vi "Arcade Drive Translate.vi"(8 "xAxis":dbl, 9 "yAxis":dbl) -> (1 "outputX":dbl, 2 "outputY":dbl)   [LabVIEW 2015]
uses:
  Global Ref.vi
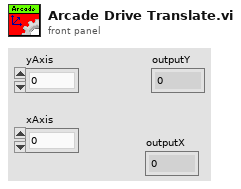
[diagram p1: front panel]
types:
  T1 = typedef "Global Ref typedef.ctl" = cluster{"Drive":cluster{"RobotDriveDevRef":T2}, "Joysticks":cluster{"JoyDriveRef":T10, "JoyOpRef":T10, "JoySabatourRef":T10}, "Lift":cluster{"LiftMotorRefLeft":T3, "LiftMotorRefRight":T3}, "Lift Limits":cluster{"Bottom Left":T12, "Bottom Right":T12}, "Accel":cluster{"AccelerometerDevRef":T14}, "Lift Encoder":cluster{"AIDeviceRefRight":T22, "AIDeviceRefLeft":T22}, "Lights":cluster{"Swag Light Ref cluster":cluster{"PWMDeviceRef1":T23, "PWMDeviceRef2":T23, "PWMDeviceRef3":T23, "PWMDeviceRef4":T23, "PWMDeviceRef5":T23, "PWMDeviceRef6":T23, "PWMDeviceRef7":T23, "PWMDeviceRef8":T23}}, "Camera":cluster{"GrayScaleImage":T24, "ColorImage":T24, "CameraDevRef":T25}, "Drive Encoders":cluster{"AIDeviceRef Left":T22, "AIDeviceRef Right":T22}, "Gyro":cluster{"GyroDevRef":T26}, "Relay":cluster{"RelayDevRef":T27, "RelayDevRef 2":T27}, "Gripper Arm Motors":cluster{"Gripper Arm Left":T3, "Gripper Arm Right":T3}, "Gripper Arm Limit":cluster{"Gripper Arm Left":T12, "Gripper Arm Right":T12}}
  T2 = typedef "WPI_RobotDriveDevRef.ctl" = cluster{"DevStatus":errorcluster, "Motors[]":T3[], "Square Inputs":bool, "Max Output":dbl}
  T3 = typedef "WPI_MotorControlDeviceRef.ctl" = cluster{"DeviceStatus":errorcluster, "Type":T4, "PWM":cluster{"PWM Channel":T5, "DeadBand":T6}, "CAN":cluster{"Device Number":u8, "Control Mode":T7, "Semaphore":T8, "Max Vout":dbl, "TalonSRX Control Mode":T9}, "Invert":bool}
  T4 = typedef "WPI_MotorControlType.ctl" = enum16{"PWM", "CAN", "CANTalonSRX"}
  T5 = typedef "FPGA_DIOPWMChannel.ctl" = enum8{"PWM 0", "PWM 1", "PWM 2", "PWM 3", "PWM 4", "PWM 5", "PWM 6", "PWM 7", "PWM 8", "PWM 9", "PWM MXP 0", "PWM MXP 1", "PWM MXP 2", "PWM MXP 3", "PWM MXP 4", "PWM MXP 5", "PWM MXP 6", "PWM MXP 7", "PWM MXP 8", "PWM MXP 9", "Invalid"}
  T6 = typedef "WPI_PWMDeadband.ctl" = cluster{"Name":string, "maxPositivePwm":i32, "minPositivePwm":i32, "centerPwm":i32, "maxNegativePwm":i32, "minNegativePwm":i32, "angularRange":u16}
  T7 = typedef "WPI_CANJaguar_ControlMode.ctl" = enum8{"Percent VBus", "Current", "Speed", "Position", "Voltage"}
  T8 = typedef "Semaphore RefNum" = refnum<k1>
  T9 = typedef "WPI_CANTalonSRX_APIControlMode.ctl" = enum8{"Percent VBus", "Speed", "Position", "Slave", "Unchanged / Invalid", "Voltage Compensation", "Current", "Motion Profile"}
  T10 = typedef "WPI_JoystickDevRef.ctl" = cluster{"Device":T11}
  T11 = typedef "WPI_JoystickDeviceEnum.ctl" = enum16{"USB 0", "USB 1", "USB 2", "USB 3", "USB 4", "USB 5"}
  T12 = typedef "WPI_DigitalInputDevRef.ctl" = cluster{"DevStatus":errorcluster, "DIO Channel":T13}
  T13 = typedef "FPGA_DIOChannel.ctl" = enum8{"DIO 0", "DIO 1", "DIO 2", "DIO 3", "DIO 4", "DIO 5", "DIO 6", "DIO 7", "DIO 8", "DIO 9", "DIO MXP 0", "DIO MXP 1", "DIO MXP 2", "DIO MXP 3", "DIO MXP 4", "DIO MXP 5", "DIO MXP 6", "DIO MXP 7", "DIO MXP 8", "DIO MXP 9", "DIO MXP 10", "DIO MXP 11", "DIO MXP 12", "DIO MXP 13", "DIO MXP 14", "DIO MXP 15", "Invalid"}
  T14 = typedef "WPI_AccelerometerDevRef.ctl" = cluster{"DevStatus":errorcluster, "Scaling":T15, "Analog Channels":T16, "I2C Bus":T18, "SPI Bus":T19, "Accel Range":T20, "ADXL Axes":T21, "Handle":i32, "Device Address":u8, "Accel Type":enum16{"Analog", "ADXL345 I2C", "ADXL345 SPI", "Internal", "ADXL362 SPI"}}
  T15 = typedef "WPI_AccelerometerScaling.ctl" = cluster{"Gain (VoltsPerG)":dbl, "Center Voltage":dbl}
  T16 = typedef "WPI_AccelerometerAnalogChannels.ctl" = cluster{"X-Axis":T17, "Y-Axis":T17, "Z-Axis":T17}
  T17 = typedef "FPGA_AIChannel.ctl" = enum8{"AI 0", "AI 1", "AI 2", "AI 3", "AI MXP 0", "AI MXP 1", "AI MXP 2", "AI MXP 3", "Invalid"}
  T18 = typedef "i2c_bus.ctl" = enum16{"I2C On-Board", "I2C MXP", "Invalid"}
  T19 = typedef "spi_bus.ctl" = enum16{"SPI On-Board, CS0", "SPI On-Board, CS1", "SPI On-Board, CS2", "SPI On-Board, CS3", "SPI MXP", "Invalid"}
  T20 = typedef "ADXL345 Range.ctl" = u8
  T21 = typedef "WPI_AccelerometerADXL345 Axes.ctl" = cluster{"X-Axis":bool, "Y-Axis":bool, "Z-Axis":bool}
  T22 = typedef "WPI_AnalogChannelDevRef.ctl" = cluster{"DevStatus":errorcluster, "Analog Channel":T17}
  T23 = typedef "WPI_PWMDeviceRef.ctl" = cluster{"DeviceStatus":errorcluster, "PWM Channel":T5}
  T24 = typedef "IMAQ Image.ctl" = refnum<image>
  T25 = typedef "WPI_CameraDevRef.ctl" = cluster{"Camera Address":string, "CameraStatus":errorcluster}
  T26 = typedef "WPI_GyroDevRef.ctl" = cluster{"DevStatus":errorcluster, "Analog Channel":T17, "Offset":dbl, "Gain (VoltsPerDegree/Second)":dbl, "Gyro Type":enum16{"Analog", "XRS450"}, "Handle":i32, "SPI Bus":T19, "Device Found":bool, "Sample Rate":dbl, "Calibrate On Open":bool}
  T27 = typedef "WPI_RelayDevRef.ctl" = cluster{"DevStatus":errorcluster, "Relay Channel":T28, "Relay Direction":T29}
  T28 = typedef "FPGA_DIORelayChannel.ctl" = enum8{"Relay 0", "Relay 1", "Relay 2", "Relay 3", "Invalid"}
  T29 = typedef "WPI_RelayDirection.ctl" = enum16{"Both directions", "Forward only", "Reverse only"}
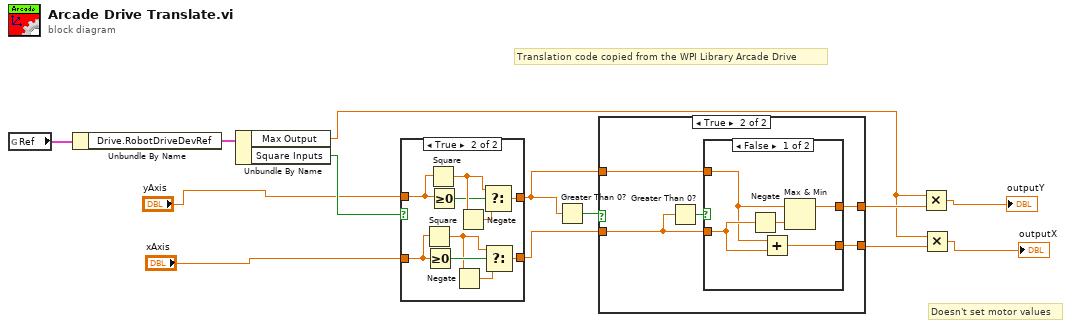
[diagram p0: block diagram]
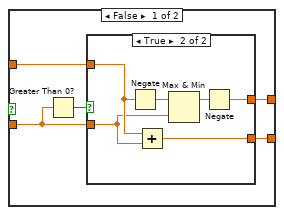
[diagram p2: hidden frame]
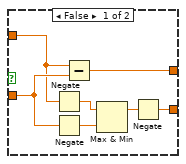
[diagram p3: hidden frame]
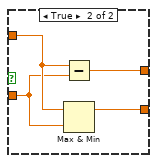
[diagram p4: hidden frame]
diagram:
  # "Doesn't set motor values"
  # "Translation code copied from the WPI Library Arcade Drive"
  n1 = global read "Global Ref.vi" "Ref"() -> (w13:T1)
  n2 = Unbundle By Name(w13) -> ("Drive.RobotDriveDevRef"=w12:T2)
  n3 = Unbundle By Name(w12) -> ("Max Output"=w5:dbl, "Square Inputs"=w11:bool)
  n4 = case shown="True" w11 {
    tunnel: [w14 w25] -> w10
    tunnel: [w15 w24] -> w8
    tunnel: "xAxis" -> [w14 w23]
    tunnel: "yAxis" -> [w15 w22]
    frame False {
    }
    frame True {
      n5 = Square(x=w23) -> (x^2=w20:dbl)
      n6 = Greater Or Equal To 0?(x=w23) -> (x >= 0?=w21:bool)
      n7 = Square(x=w22) -> (x^2=w17:dbl)
      n8 = Greater Or Equal To 0?(x=w22) -> (x >= 0?=w16:bool)
      n9 = Negate(x=w20) -> (-x=w19:dbl)
      n10 = Negate(x=w17) -> (-x=w18:dbl)
      n11 = Select(t=w17, s=w16, f=w18) -> (s? t:f=w24:dbl)
      n12 = Select(t=w20, s=w21, f=w19) -> (s? t:f=w25:dbl)
    }
  }
  n13 = Greater Than 0?(x=w8) -> (x > 0?=w9:bool)
  n14 = case shown="True" w9 {
    tunnel: w10 -> [w29 w47]
    tunnel: w8 -> [w28 w46]
    tunnel: [w27 w45] -> w6
    tunnel: [w26 w44] -> w7
    frame False {
      n15 = Greater Than 0?(x=w29) -> (x > 0?=w30:bool)
      n16 = case shown="True" w30 {
        tunnel: w29 -> [w37 w39]
        tunnel: w28 -> [w35 w40]
        tunnel: [w31 w41] -> w27
        tunnel: [w32 w38] -> w26
        frame False {
          n17 = Negate(x=w35) -> (-x=w36:dbl)
          n18 = Negate(x=w37) -> (-x=w34:dbl)
          n19 = Subtract(x=w35, y=w37) -> (x-y=w31:dbl)
          n20 = Max & Min(x=w36, y=w34) -> (max(x,y)=w33:dbl)  [unwired: 1 out]
          n21 = Negate(x=w33) -> (-x=w32:dbl)
        }
        frame True {
          n22 = Negate(x=w40) -> (-x=w43:dbl)
          n23 = Add(x=w40, y=w39) -> (x+y=w38:dbl)
          n24 = Max & Min(x=w43, y=w39) -> (max(x,y)=w42:dbl)  [unwired: 1 out]
          n25 = Negate(x=w42) -> (-x=w41:dbl)
        }
      }
    }
    frame True {
      n26 = Greater Than 0?(x=w47) -> (x > 0?=w48:bool)
      n27 = case shown="False" w48 {
        tunnel: w47 -> [w53 w55]
        tunnel: w46 -> [w50 w56]
        tunnel: [w51 w54] -> w45
        tunnel: [w49 w57] -> w44
        frame False {
          n28 = Negate(x=w53) -> (-x=w52:dbl)
          n29 = Add(x=w50, y=w53) -> (x+y=w49:dbl)
          n30 = Max & Min(x=w50, y=w52) -> (max(x,y)=w51:dbl)  [unwired: 1 out]
        }
        frame True {
          n31 = Subtract(x=w56, y=w55) -> (x-y=w54:dbl)
          n32 = Max & Min(x=w56, y=w55) -> (max(x,y)=w57:dbl)  [unwired: 1 out]
        }
      }
    }
  }
  n33 = Multiply(x=w5, y=w6) -> (x*y=→"outputY":dbl)
  n34 = Multiply(x=w5, y=w7) -> (x*y=→"outputX":dbl)
